vi "aughit.vi"() -> ()   [LabVIEW 2013]
uses:
  <vilib>/Analysis/NI_AALPro.lvlib
  <vilib>/imath/engines/lvmath2/RunTimeEngine/RunTimeType/NIMS_RunTimeType_From StrictType (excl LVString).vi
  <vilib>/imath/engines/lvmath2/RunTimeEngine/Struct/NIMS_StructSetField.vi
  <vilib>/imath/engines/lvmath2/RunTimeEngine/RangeToken/NIMS_Range.vi
  <vilib>/imathl/engines/lvmath/Functions/Error Handling/Create Error.vi
  <vilib>/imath/engines/lvmath2/RunTimeEngine/RangeToken/NIMS_Range_R2 - Integer.vi
  <vilib>/imath/engines/lvmath2/RunTimeEngine/IndexRead/NIMS V(S).vi
  <vilib>/imath/engines/lvmath2/RunTimeEngine/Struct/NIMS_StructGetField.vi
  <vilib>/imath/engines/lvmath2/RunTimeEngine/RunTimeType/NIMS_RunTimeType_To Numeric.vi
  <vilib>/imath/engines/lvmath2/RunTimeEngine/VariableToken/NIMS_VariableToken_CondDefinedDefinedByReplace.vi
  <vilib>/imath/engines/lvmath2/RunTimeEngine/IndexReplace/NIMS V(S)=S.vi
  <vilib>/imath/engines/lvmath2/RunTimeEngine/ErrorHandling/NIMS_Create Error From Enums.vi
  <vilib>/imath/engines/lvmath2/RunTimeEngine/CommandStatement/MC_CommandStatement_break.vi
  <vilib>/imath/engines/lvmath2/RunTimeEngine/NodeEndStatement/NIMS_NodeEndStatement_Output.vi
  <vilib>/imath/engines/lvmath2/RunTimeEngine/ErrorHandling/NIMS_Finalize Error.vi
panel:
  out "Matches (Color Pattern Matching 2)":T1(array[cluster]) {"Bounding Box"."y" format="%.2f"; "Bounding Box"."x" format="%.2f"; "Position"."y" format="%.2f"; "Position"."x" format="%.2f"; "Score" format="%.2f"; "Scale" format="%.2f"; "Angle" format="%.2f"}
  out "Array":T2(array[cluster])
  out "XY Graph 2":cluster{"x":dbl[], "y":dbl[]}(graph)
  out "y2":sgl[](array[numeric])
  out "x2":sgl[](array[numeric])
  out "XY Graph":cluster{"Y":dbl[], "Y":dbl[]}[](graph)
  out "x":sgl
  out "y":sgl
  out "appended array":sgl[](array[numeric])
  out "Image Out 2":T3(plugin-control)
  in  "Stop (F)":bool
  out "Image Out":T3(plugin-control)
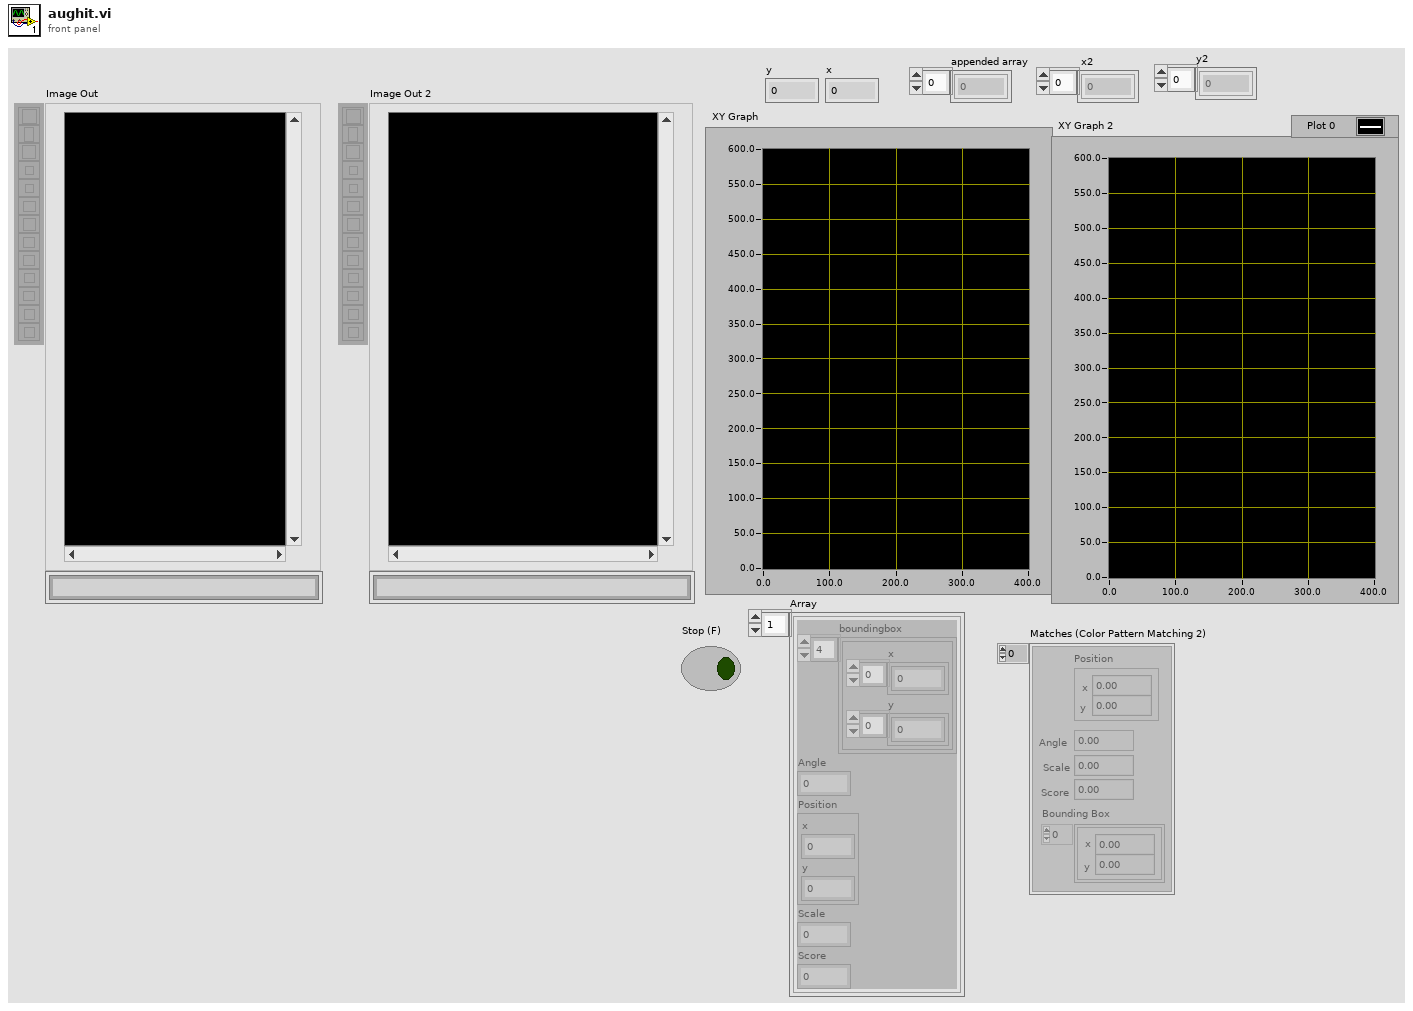
[diagram p1: front panel]
types:
  T1 = cluster{"Position":cluster{"x":sgl, "y":sgl}, "Angle":sgl, "Scale":sgl, "Score":sgl, "Bounding Box":cluster{"x":sgl, "y":sgl}[]}[]
  T2 = cluster{"boundingbox":cluster{"x":sgl[], "y":sgl[]}[], "Angle":sgl, "Position":cluster{"x":sgl, "y":sgl}, "Scale":sgl, "Score":sgl}[]
  T3 = typedef "IMAQ Image.ctl" = refnum<image>
  T4 = cluster{"Position":cluster{"x":sgl, "y":sgl}, "Angle":sgl, "Scale":sgl, "Score":sgl, "Bounding Box":cluster{"x":sgl, "y":sgl}[]}
  T5 = cluster{"Bounding Box[0]":cluster{"x":sgl, "y":sgl}, "Bounding Box[1]":cluster{"x":sgl, "y":sgl}, "Bounding Box[2]":cluster{"x":sgl, "y":sgl}, "Bounding Box[3]":cluster{"x":sgl, "y":sgl}}
  T6 = cluster{"[0]":sgl, "[1]":sgl, "[2]":sgl, "[3]":sgl}
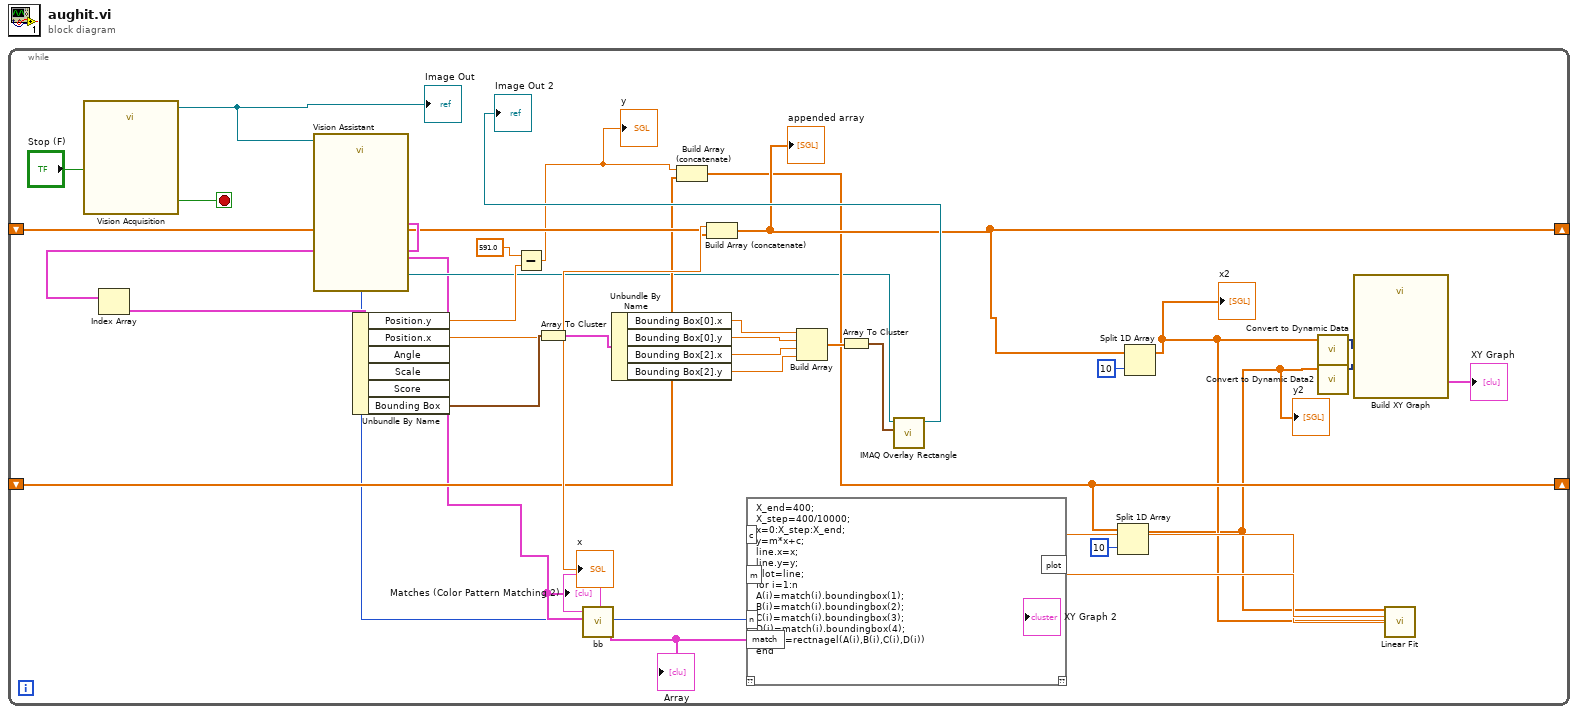
[diagram p0: block diagram]
diagram:
  n1 = while {
    shift-right: [w14] -> _
    shift-left: _ -> [w21]
    shift-right: [w13] -> _
    shift-left: _ -> [w20]
    stop <- w35 stop-if-true
    n2 = call "Vision Acquisition"("Stop (F)"="Stop (F)") -> ("Image Out"=w34:T3, "Stopped"=w35:bool)  [unwired: 24 in, 1 out]
    "Image Out" <- w34
    n3 = call "Vision Assistant"("Image In"=w34) -> ("Image Out"=w4:T3, "Matches (Color Pattern Matching 1)"=w33:T1, "Number of Matches (Color Pattern Matching 2)"=w1:i32, "Matches (Color Pattern Matching 2)"=w3:T1)  [unwired: 22 in, 1 out]
    "Matches (Color Pattern Matching 2)" <- w3
    n4 = Index Array(array=w33) -> (element=w32:T4)  [unwired: 1 in]
    n5 = Unbundle By Name(w32) -> ("Position.y"=w19:sgl, "Position.x"=w22:sgl, "Bounding Box"=w31:cluster{"x":sgl, "y":sgl}[])  [unwired: 3 out]
    "x" <- w22
    n6 = Subtract(x=sgl 591.0, y=w19) -> (x-y=w10:sgl)
    "y" <- w10
    n7 = Array To Cluster(array=w31) -> (cluster=w30:T5)
    n8 = call "bb.vi"("Matches (Color Pattern Matching 2)"=w3) -> ("Array"=w2:T2)  [unwired: 10 in]
    "Array" <- w2
    n9 = Unbundle By Name(w30) -> ("Bounding Box[0].x"=w29:sgl, "Bounding Box[0].y"=w28:sgl, "Bounding Box[2].x"=w27:sgl, "Bounding Box[2].y"=w26:sgl)
    n10 = Build Array (concatenate)(w10, w20) -> (w13:sgl[])
    n11 = Build Array (concatenate)(w22, w21) -> (w14:sgl[])
    "appended array" <- w14
    n12 = Build Array(w29, w28, w27, w26) -> (w25:sgl[])
    n13 = Array To Cluster(array=w25) -> (cluster=w24:T6)
    n14 = call "IMAQ Overlay Rectangle"("Rectangle"=w24, "Image"=w4) -> ("Image Out"=→"Image Out 2":T3)  [unwired: 8 in, 1 out]
    n15 = Split 1D Array(array=w13, index=10) -> (first subarray=w5:sgl[])  [unwired: 1 out]
    "y2" <- w5
    n16 = Split 1D Array(array=w14, index=10) -> (first subarray=w6:sgl[])  [unwired: 1 out]
    "x2" <- w6
    n17 = call "Convert to Dynamic Data"("Array"=w6) -> ("Dynamic Data Type"=w16:dynamicdata)  [unwired: 3 in]
    n18 = call "Convert to Dynamic Data2"("Array"=w5) -> ("Dynamic Data Type"=w15:dynamicdata)  [unwired: 3 in]
    n19 = call "Build XY Graph"("Y Input"=w15, "X Input"=w16) -> ("XY Graph"=→"XY Graph":cluster{"X":dbl[], "Y":dbl[]}[])  [unwired: 8 in, 1 out]
    n20 = call <vilib>:"Linear Fit.vi"("Y"=w5, "X"=w6) -> ("slope"=w9:dbl, "intercept"=w8:dbl)  [unwired: 9 in, 3 out]
    n21 = mathscript code="X_end=400;\nX_step=400/10000;\nx=0:X_step:X_end;\ny=m*x+c;\nline.x=x;\nline.y=y;\nplot=line;\nfor i=1:n\nA(i)=match(i).boundingbox(1);\nB(i)=match(i).boundingbox(2);\nC(i)=match(i).boundingbox(3);\nD(i)=match(i).boundingbox(4);\nline(i)=rectnagel(A(i),B(i),C(i),D(i))\nend"("c"=w8, "m"=w9, "match"=w2, "n"=w1) -> ("plot"=→"XY Graph 2":cluster{"x":dbl[], "y":dbl[]})  [unwired: 1 in, 1 out]
  }
